vi "RPED Globals.vi"() -> ()   [LabVIEW 2017]
uses:
  RPED Notifier.ctl
  RPED Control Type.ctl
panel:
  in  "RPED Cals":dbl[](array[numeric])
  in  "RPED Execute Notifier":refnum<notifier>
  in  "RPED Set Notifier":refnum<notifier>
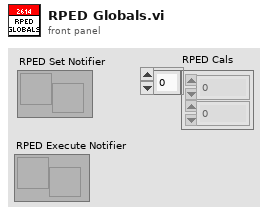
[diagram p1: front panel]
diagram:
